vi "XML to Experimental Parameters.vi"(0 "XML Data":string) -> ()   [LabVIEW 2013]
uses:
  Types/Experimental Parameters.ctl
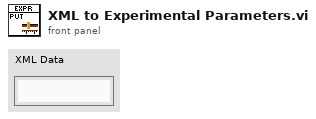
[diagram p1: front panel]
types:
  T1 = typedef "Experimental Parameters.ctl" = cluster{"Number of Samples":dbl, "Ramp Rate":dbl, "Version":string}
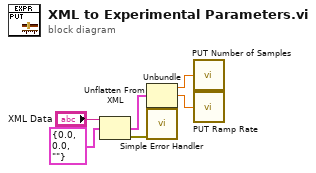
[diagram p0: block diagram]
diagram:
  n1 = Unflatten From XML(xml string="XML Data", type=T1 {"Number of Samples"=0.0, "Ramp Rate"=0.0, "Version"=""} ("Experimental Parameters")) -> (value=w3:T1, error out=w6:errorcluster)  [unwired: 1 in]
  n2 = Unbundle(w3) -> ("Number of Samples"=w2:dbl, "Ramp Rate"=w1:dbl)  [unwired: 1 out]
  n3 = call <vilib>:"Simple Error Handler.vi"("error in (no error)"=w6) -> ()  [unwired: 4 in, 5 out]
  n4 = call "PUT Number of Samples.vi"("Number of Samples"=w2) -> ()
  n5 = call "PUT Ramp Rate.vi"("Ramp Rate"=w1) -> ()
